vi "Example_Simple_Plot.vi"() -> ()   [LabVIEW 2020]
panel:
  out "Angular Speed Motor":cluster{"OmegaR":dbl, "OmegaL":dbl}(graph)
  out "SonarDistance":dbl
  in  "ServoAngle":dbl
  in  "ControlR (-1 to 1)":dbl min=-1.0 max=1.0 step=0.01
  in  "IP Address":string="192.168.1.1"
  in  "Mode Select":T1(ring)
  out "Velocity Right":dbl
  out "Velocity Left":dbl
  in  "dt (ms)":u32=10
  in  "ControlL (-1 to 1)":dbl min=-1.0 max=1.0 step=0.01
  in  "stop":bool
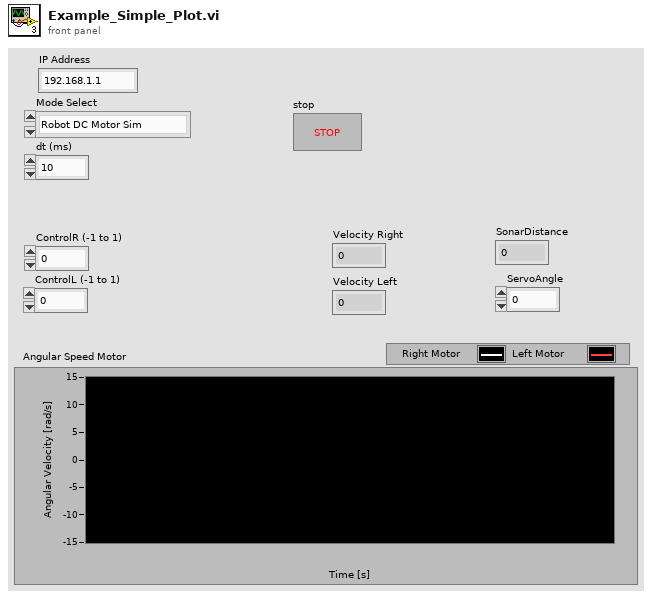
[diagram p1: front panel]
types:
  T1 = enum16{"Robot DC Motor Sim", "Robot Simulation", "Real Robot"}
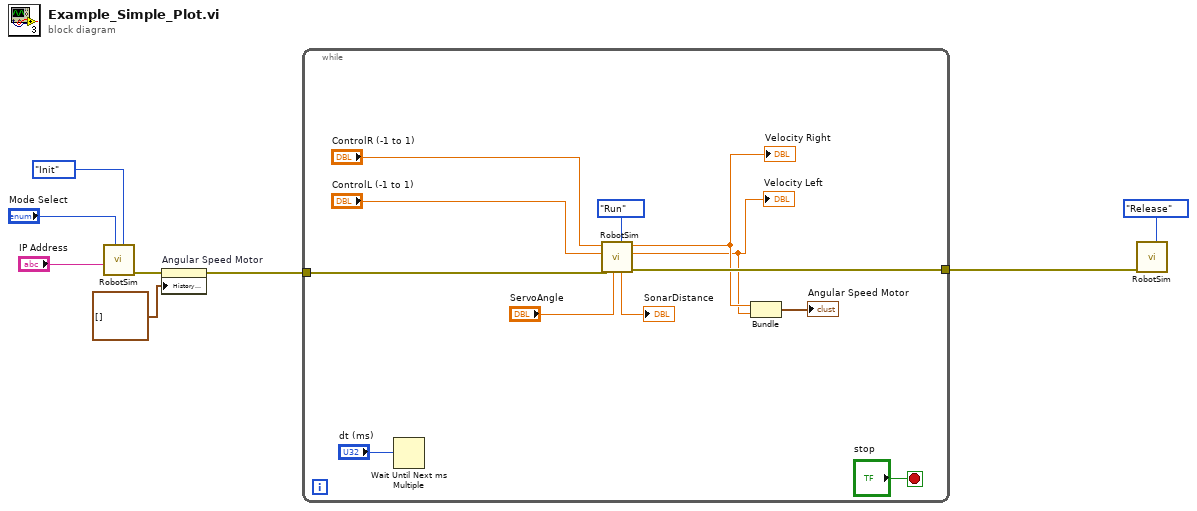
[diagram p0: block diagram]
diagram:
  n1 = call "RobotSim.vi"("Action"=enum16{"Init", "Run", "Release"}."Init", "Mode Select"="Mode Select", "IP Address"="IP Address") -> ("error out"=w3:errorcluster)  [unwired: 4 in, 4 out]
  n2 = property on="Angular Speed Motor" class="WFChart (strict)"(error in=w3, "History Data"=cluster{"OmegaR":dbl, "OmegaL":dbl}[] []) -> (error out=w1:errorcluster)  [unwired: 1 in, 1 out]
  n3 = while {
    tunnel: [w18] -> w7
    tunnel: w1 -> [w10]
    stop <- "stop" stop-if-true
    n4 = Wait Until Next ms Multiple(millisecond multiple="dt (ms)") -> ()  [unwired: 1 out]
    n5 = call "RobotSim.vi"("Action"=enum16{"Init", "Run", "Release"}."Run", "ServoAngle"="ServoAngle", "error in (no error)"=w10, "ControlL"="ControlL (-1 to 1)", "ControlR"="ControlR (-1 to 1)") -> ("error out"=w18:errorcluster, "OmegaL"=w12:dbl, "OmegaR"=w13:dbl, "SonarDistance"=→"SonarDistance":dbl)  [unwired: 2 in, 1 out]
    "Velocity Left" <- w12
    "Velocity Right" <- w13
    n6 = Bundle("OmegaR"=w13, "OmegaL"=w12) -> (→"Angular Speed Motor":cluster{"OmegaR":dbl, "OmegaL":dbl})  [unwired: 1 in]
  }
  n7 = call "RobotSim.vi"("Action"=enum16{"Init", "Run", "Release"}."Release", "error in (no error)"=w7) -> ()  [unwired: 5 in, 5 out]
